vi "MAIN-Backup.vi"(6 "ECU TYPE":u16(ring) items=["LSMD", "LSMP", "LSMRL", "LSMRR"]) -> (0 "Data By ID OK":bool, 1 "Hall Test 3 OK":bool, 2 "Sleep Request OK":bool, 3 "Hall Test 1 OK":bool, 4 "SBC OK":bool, 5 "Hall Test 2 OK":bool, 7 "Hard Reset OK":bool, 8 "BIST OK":bool, 9 "SW Version OK":bool, 10 "ECU ID OK":bool, 11 "Session OK":bool)   [LabVIEW 2022 SP3]
uses:
  USB 8502/Sub VIs/Global .vi
panel:
  out "Enter Brose Ext OK":bool
  out "Hall Test 3 Response":string
  out "Enter Brose Ext":string
  out "ECU Hard Reset":string
  out "Program SBC":string
  out "ID Response":string
  out "ID Request":string
  out "Tester Present OK":bool
  out "Hall Test 2 Response":string
  out "Hall Test 1 Response":string
  out "Supply Voltage ADC Response":string
  out "Self Test BIST":string
  out "Sleep Request Response":string
  out "Read Data By ID":string
  out "Verify ECU ID String":string
  out "Verify SW Version":string
  out "Tester Present Command":string
  out "Enter Brose EOL Ext Session":string
  # "*Revisar debido a cambio en respuesta"
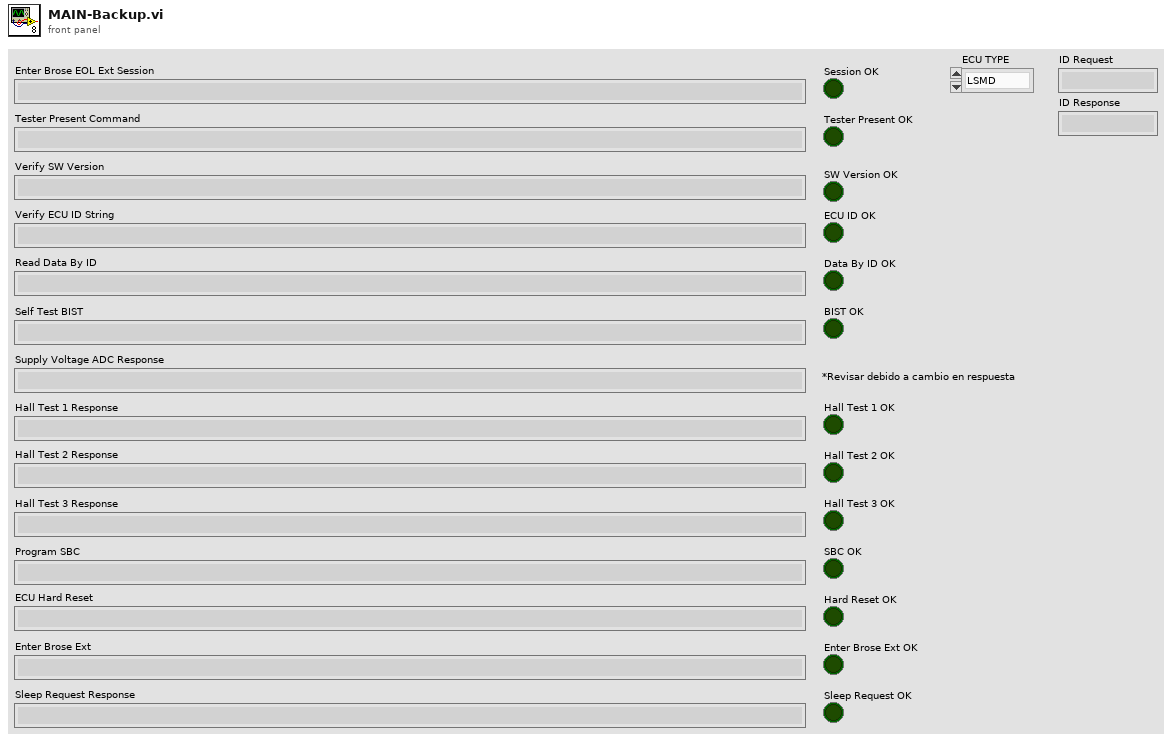
[diagram p1: front panel]
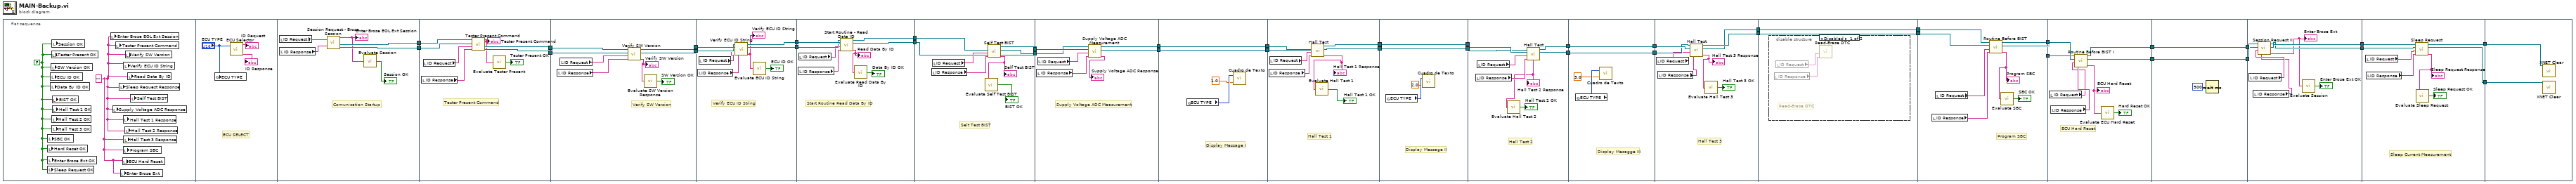
[diagram p0: block diagram]
diagram:
  n1 = flat-sequence {
    tunnel: [w49] -> w38
    tunnel: [w48] -> w37
    tunnel: w38 -> [w57]
    tunnel: w37 -> [w56]
    tunnel: [w55] -> w32
    tunnel: [w54] -> w31
    tunnel: [w62] -> w34
    tunnel: [w63] -> w33
    tunnel: w32 -> [w65]
    tunnel: w31 -> [w64]
    tunnel: [w70] -> w36
    tunnel: [w71] -> w35
    tunnel: w34 -> [w73]
    tunnel: w33 -> [w72]
    tunnel: [w79] -> w30
    tunnel: [w78] -> w29
    tunnel: w36 -> [w81]
    tunnel: w35 -> [w80]
    tunnel: [w85] -> w28
    tunnel: [w84] -> w27
    tunnel: w29 -> [w86]
    tunnel: w30 -> [w87]
    tunnel: [w96] -> w2
    tunnel: [w95] -> w1
    tunnel: w28 -> [w91]
    tunnel: w27 -> [w90]
    tunnel: [w100] -> w12
    tunnel: [w99] -> w11
    tunnel: w1 -> [w99]
    tunnel: w2 -> [w100]
    tunnel: w12 -> [w108]
    tunnel: w11 -> [w107]
    tunnel: [w106] -> w10
    tunnel: [w105] -> w8
    tunnel: w10 -> [w112]
    tunnel: [w112] -> w9
    tunnel: w8 -> [w111]
    tunnel: [w111] -> w7
    tunnel: w9 -> [w120]
    tunnel: w7 -> [w119]
    tunnel: [w118] -> w6
    tunnel: [w117] -> w4
    tunnel: w6 -> [w124]
    tunnel: [w124] -> w5
    tunnel: w4 -> [w123]
    tunnel: [w123] -> w3
    tunnel: w5 -> [w131]
    tunnel: w3 -> [w132]
    tunnel: [w130] -> w15
    tunnel: [w129] -> w13
    tunnel: [w134] -> w16
    tunnel: w15 -> [w134]
    tunnel: [w133] -> w14
    tunnel: w13 -> [w133]
    tunnel: [w142] -> w26
    tunnel: [w141] -> w25
    tunnel: w16 -> [w140]
    tunnel: w14 -> [w139]
    tunnel: w26 -> [w150]
    tunnel: w25 -> [w149]
    tunnel: [w148] -> w20
    tunnel: [w147] -> w18
    tunnel: w20 -> [w155]
    tunnel: [w155] -> w19
    tunnel: w18 -> [w154]
    tunnel: [w154] -> w17
    tunnel: w19 -> [w163]
    tunnel: w17 -> [w162]
    tunnel: [w159] -> w22
    tunnel: [w158] -> w21
    tunnel: [w169] -> w24
    tunnel: [w168] -> w23
    tunnel: w22 -> [w167]
    tunnel: w21 -> [w166]
    tunnel: w24 -> [w173]
    tunnel: w23 -> [w172]
    frame #0 {
      w39 = FALSE
      w40 = ""
      n2 = local write "Hard Reset OK"(w39) -> ()
      n3 = local write "Sleep Request OK"(w39) -> ()
      n4 = local write "SBC OK"(w39) -> ()
      n5 = local write "Enter Brose Ext OK"(w39) -> ()
      n6 = local write "ECU ID OK"(w39) -> ()
      n7 = local write "Data By ID OK"(w39) -> ()
      n8 = local write "SW Version OK"(w39) -> ()
      n9 = local write "Tester Present OK"(w39) -> ()
      n10 = local write "Session OK"(w39) -> ()
      n11 = local write "Hall Test 2 OK"(w39) -> ()
      n12 = local write "Hall Test 3 OK"(w39) -> ()
      n13 = local write "BIST OK"(w39) -> ()
      n14 = local write "Hall Test 1 OK"(w39) -> ()
      n15 = local write "Enter Brose EOL Ext Session"(w40) -> ()
      n16 = local write "Supply Voltage ADC Response"(w40) -> ()
      n17 = local write "Tester Present Command"(w40) -> ()
      n18 = local write "Sleep Request Response"(w40) -> ()
      n19 = local write "Enter Brose Ext"(w40) -> ()
      n20 = local write "ECU Hard Reset"(w40) -> ()
      n21 = local write "Hall Test 1 Response"(w40) -> ()
      n22 = local write "Program SBC"(w40) -> ()
      n23 = local write "Verify ECU ID String"(w40) -> ()
      n24 = local write "Hall Test 3 Response"(w40) -> ()
      n25 = local write "Hall Test 2 Response"(w40) -> ()
      n26 = local write "Verify SW Version"(w40) -> ()
      n27 = local write "Read Data By ID"(w40) -> ()
      n28 = local write "Self Test BIST"(w40) -> ()
    }
    frame #1 {
      # "ECU SELECT"
      n29 = global write "Global .vi" "ECU TYPE"("ECU TYPE") -> ()
      n30 = call "ECU Selector.vi"("ECU TYPE"="ECU TYPE") -> ("ID Request"=→"ID Request":string, "ID Response"=→"ID Response":string)  [unwired: 1 in, 2 out]
    }
    frame #2 {
      # "Comunication Startup"
      n31 = local read "ID Request"() -> (w46:string)
      n32 = local read "ID Response"() -> (w45:string)
      n33 = call "Session Request - Brose Session.vi"("ID Request"=w46, "ID Response"=w45) -> ("Data String"=w47:string, "Write"=w49:refnum<k21>, "Read"=w48:refnum<k21>)  [unwired: 1 out]
      "Enter Brose EOL Ext Session" <- w47
      n34 = call "Evaluate Session.vi"("String In"=w47) -> ("Test OK"=→"Session OK":bool)
    }
    frame #3 {
      # "Tester Present Command"
      n35 = local read "ID Response"() -> (w50:string)
      n36 = local read "ID Request"() -> (w51:string)
      n37 = call "Tester Present Command.vi"("ID Response"=w50, "ID Request"=w51, "Read"=w56, "Write"=w57) -> ("Read out"=w55:refnum<k21>, "Write out"=w54:refnum<k21>, "Data String 2"=w53:string)  [unwired: 1 out]
      "Tester Present Command" <- w53
      n38 = call "Evaluate Tester Present.vi"("String In"=w53) -> ("Test OK"=→"Tester Present OK":bool)
    }
    frame #4 {
      # "Verify SW Version"
      n39 = local read "ID Response"() -> (w58:string)
      n40 = local read "ID Request"() -> (w59:string)
      n41 = call "Verify SW Version.vi"("ID Response"=w58, "ID Request"=w59, "Read"=w65, "Write"=w64) -> ("Data String 3"=w61:string, "Write out"=w63:refnum<k21>, "Read out"=w62:refnum<k21>)  [unwired: 1 out]
      "Verify SW Version" <- w61
      n42 = call "Evaluate SW Version Response.vi"("String In"=w61) -> ("Test OK"=→"SW Version OK":bool)
    }
    frame #5 {
      # "Verify ECU ID String"
      n43 = local read "ID Response"() -> (w68:string)
      n44 = local read "ID Request"() -> (w69:string)
      n45 = call "Verify ECU ID String.vi"("ID Response"=w68, "ID Request"=w69, "Read"=w73, "Write"=w72) -> ("Data String 3"=w67:string, "Write out"=w71:refnum<k21>, "Read out"=w70:refnum<k21>)  [unwired: 1 out]
      "Verify ECU ID String" <- w67
      n46 = call "Evaluate ECU ID String.vi"("String In"=w67) -> ("Test OK"=→"ECU ID OK":bool)
    }
    frame #6 {
      # "Start Routine Read Data By ID"
      n47 = local read "ID Response"() -> (w76:string)
      n48 = local read "ID Request"() -> (w77:string)
      n49 = call "Start Routine - Read Data ID.vi"("ID Response"=w76, "ID Request"=w77, "Read"=w81, "Write"=w80) -> ("Data String 3"=w75:string, "Write out"=w79:refnum<k21>, "Read out"=w78:refnum<k21>)  [unwired: 1 out]
      "Read Data By ID" <- w75
      n50 = call "Evaluate Read Data By ID.vi"("String In"=w75) -> ("Test OK"=→"Data By ID OK":bool)
    }
    frame #7 {
      # "Selt Test BIST"
      n51 = local read "ID Response"() -> (w88:string)
      n52 = local read "ID Request"() -> (w89:string)
      n53 = call "Self Test BIST.vi"("ID Response"=w88, "ID Request"=w89, "Read"=w86, "Write"=w87) -> ("Data String 3"=w82:string, "Write out"=w84:refnum<k21>, "Read out"=w85:refnum<k21>)  [unwired: 1 out]
      "Self Test BIST" <- w82
      n54 = call "Evaluate Self Test BIST.vi"("String In"=w82) -> ("Test OK"=→"BIST OK":bool)
    }
    frame #8 {
      # "Supply Voltage ADC Measurement"
      n55 = local read "ID Response"() -> (w92:string)
      n56 = local read "ID Request"() -> (w93:string)
      n57 = call "Supply Voltage ADC Measurement.vi"("ID Response"=w92, "ID Request"=w93, "Read"=w91, "Write"=w90) -> ("Data String 3"=→"Supply Voltage ADC Response":string, "Write out"=w96:refnum<k21>, "Read out"=w95:refnum<k21>)  [unwired: 1 out]
    }
    frame #9 {
      # "Display Message I"
      n58 = global read "Global .vi" "ECU TYPE"() -> (w98:u16)
      n59 = call "Cuadro de Texto.vi"("Numeric"=1.0, "ECU TYPE"=w98) -> ()  [unwired: 2 in]
    }
    frame #10 {
      # "Hall Test 1"
      n60 = local read "ID Response"() -> (w103:string)
      n61 = local read "ID Request"() -> (w104:string)
      n62 = call "Hall Test.vi"("ID Response"=w103, "ID Request"=w104, "Read"=w107, "Write"=w108) -> ("Data String 3"=w102:string, "Write out"=w105:refnum<k21>, "Read out"=w106:refnum<k21>)  [unwired: 1 out]
      "Hall Test 1 Response" <- w102
      n63 = call "Evaluate Hall Test 1.vi"("String In"=w102) -> ("Test OK"=→"Hall Test 1 OK":bool)
    }
    frame #11 {
      # "Display Message II"
      n64 = global read "Global .vi" "ECU TYPE"() -> (w110:u16)
      n65 = call "Cuadro de Texto.vi"("Numeric"=2.0, "ECU TYPE"=w110) -> ()  [unwired: 2 in]
    }
    frame #12 {
      # "Hall Test 2"
      n66 = local read "ID Response"() -> (w115:string)
      n67 = local read "ID Request"() -> (w116:string)
      n68 = call "Hall Test.vi"("ID Response"=w115, "ID Request"=w116, "Read"=w120, "Write"=w119) -> ("Data String 3"=w114:string, "Write out"=w118:refnum<k21>, "Read out"=w117:refnum<k21>)  [unwired: 1 out]
      "Hall Test 2 Response" <- w114
      n69 = call "Evaluate Hall Test 2.vi"("String In"=w114) -> ("Test OK"=→"Hall Test 2 OK":bool)
    }
    frame #13 {
      # "Display Mesagge III"
      n70 = global read "Global .vi" "ECU TYPE"() -> (w122:u16)
      n71 = call "Cuadro de Texto.vi"("Numeric"=3.0, "ECU TYPE"=w122) -> ()  [unwired: 2 in]
    }
    frame #14 {
      # "Hall Test 3"
      n72 = local read "ID Request"() -> (w128:string)
      n73 = local read "ID Response"() -> (w127:string)
      n74 = call "Hall Test.vi"("ID Response"=w127, "ID Request"=w128, "Read"=w132, "Write"=w131) -> ("Data String 3"=w126:string, "Write out"=w129:refnum<k21>, "Read out"=w130:refnum<k21>)  [unwired: 1 out]
      "Hall Test 3 Response" <- w126
      n75 = call "Evaluate Hall Test 3.vi"("String In"=w126) -> ("Test OK"=→"Hall Test 3 OK":bool)
    }
    frame #15 {
      n76 = disable-structure shown="Disabled" {
        frame Disabled {
          # "Read-Erase DTC"
          n77 = local read "ID Response"() -> (w135:string)
          n78 = local read "ID Request"() -> (w136:string)
          n79 = call "Read-Erase DTC.vi"("ID Response"=w135, "ID Request"=w136) -> ()  [unwired: 2 in, 4 out]
        }
        frame Enabled {
        }
      }
    }
    frame #16 {
      # "Program SBC"
      n80 = local read "ID Response"() -> (w143:string)
      n81 = local read "ID Request"() -> (w144:string)
      n82 = call "Routine Before BIST.vi"("ID Response"=w143, "ID Request"=w144, "Read"=w140, "Write"=w139) -> ("Data String 3"=w138:string, "Write out"=w141:refnum<k21>, "Read out"=w142:refnum<k21>)  [unwired: 1 out]
      "Program SBC" <- w138
      n83 = call "Evaluate SBC.vi"("String In"=w138) -> ("Test OK"=→"SBC OK":bool)
    }
    frame #17 {
      # "ECU Hard Reset"
      n84 = local read "ID Request"() -> (w151:string)
      n85 = local read "ID Response"() -> (w152:string)
      n86 = call "Routine Before BIST I.vi"("ID Response"=w152, "ID Request"=w151, "Read"=w150, "Write"=w149) -> ("Data String 3"=w146:string, "Write out"=w148:refnum<k21>, "Read out"=w147:refnum<k21>)  [unwired: 1 out]
      "ECU Hard Reset" <- w146
      n87 = call "Evaluate ECU Hard Reset.vi"("String In"=w146) -> ("Test OK"=→"Hard Reset OK":bool)
    }
    frame #18 {
      n88 = Wait (ms)(milliseconds to wait=u32 500) -> ()  [unwired: 1 out]
    }
    frame #19 {
      n89 = local read "ID Request"() -> (w161:string)
      n90 = local read "ID Response"() -> (w160:string)
      n91 = call "Session Request II.vi"("ID Response"=w160, "ID Request"=w161, "Read"=w162, "Write"=w163) -> ("Data String 3"=w157:string, "Write out"=w159:refnum<k21>, "Read out"=w158:refnum<k21>)  [unwired: 1 out]
      "Enter Brose Ext" <- w157
      n92 = call "Evaluate Session.vi"("String In"=w157) -> ("Test OK"=→"Enter Brose Ext OK":bool)
    }
    frame #20 {
      # "Sleep Current Measurement"
      n93 = local read "ID Request"() -> (w171:string)
      n94 = local read "ID Response"() -> (w170:string)
      n95 = call "Sleep Request.vi"("ID Response"=w170, "ID Resquest"=w171, "Read"=w166, "Write"=w167) -> ("Data String 3"=w165:string, "Write out"=w168:refnum<k21>, "Read out"=w169:refnum<k21>)  [unwired: 1 out]
      "Sleep Request Response" <- w165
      n96 = call "Evaluate Sleep Request.vi"("String In"=w165) -> ("Test OK"=→"Sleep Request OK":bool)
    }
    frame #21 {
      n97 = call <vilib>:"XNET Clear.vi"("session in"=w173) -> ()  [unwired: 14 in, 1 out]
      n98 = call <vilib>:"XNET Clear.vi"("session in"=w172) -> ()  [unwired: 14 in, 1 out]
    }
  }
